vi "terminate.vi"(8 "error in (no error)":errorcluster, 11 "DL090202FPGAClock in":refnum<class "ClockDL090202FPGA.lvclass">) -> (0 "error out":errorcluster, 3 "DL090202FPGAClock out":refnum<class "ClockDL090202FPGA.lvclass">)   [LabVIEW 2010, in "ClockDL090202FPGA.lvclass"]
uses:
  ClockDL090202FPGA.lvclass
  ClockDL090202FPGA.lvclass/ClockDL090202FPGA.ctl
  FPGAWrapper/GenericFPGAWrapper/GenericFPGAWrapper/GenericFPGAWrapper.lvclass
  GenericClock/GenericClock/GenericClock.lvclass
  common/classes/ErrorController/ErrorController/class_data.vi
  common/classes/ErrorController/ErrorController/ErrorController.lvclass
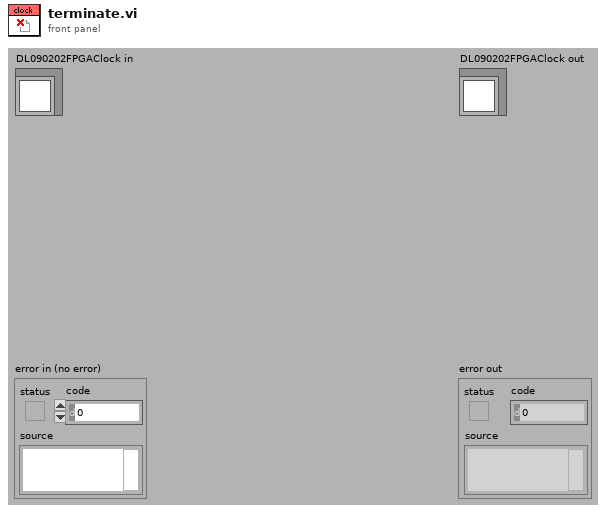
[diagram p1: front panel]
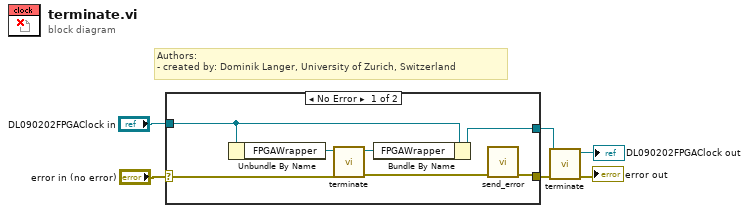
[diagram p0: block diagram]
diagram:
  # "Authors: \n- created by: Dominik Langer, University of Zurich, Switzerland"
  n1 = case shown="No Error" "error in (no error)" {
    selector: "error in (no error)" -> [w11 w15]
    tunnel: [w7 w15] -> w4
    tunnel: [w12 w14] -> w3
    tunnel: "DL090202FPGAClock in" -> [w13 w14]
    frame No Error {
      n2 = Unbundle By Name(w13) -> ("FPGAWrapper"=w10:refnum<class "GenericFPGAWrapper.lvclass">)
      n3 = call-dynamic "terminate.vi"("error in (no error)"=w11, "GenericPlugin in"=w10) -> ("error out"=w8:errorcluster, "GenericPlugin out"=w9:refnum<class "GenericFPGAWrapper.lvclass">)  [unwired: 8 out]
      n4 = Bundle By Name(cluster=w13, "FPGAWrapper"=w9) -> (w12:refnum<class "ClockDL090202FPGA.lvclass">)
      n5 = call "send_error.vi"("error in (no error)"=w8) -> ("error out"=w7:errorcluster)  [unwired: 10 in]
    }
    frame Error {
    }
  }
  n6 = call-parent "terminate.vi"("error in (no error)"=w4, "GenericPlugin in"=w3) -> ("error out"=→"error out":errorcluster, "GenericPlugin out"=→"DL090202FPGAClock out":refnum<class "ClockDL090202FPGA.lvclass">)  [unwired: 8 out]
